vi "New Edit Element.vi"(8 "error in (no error)":errorcluster, 11 "Component-B in":refnum<class "Component-B.lvclass">) -> (0 "error out":errorcluster, 3 "Component-B out":refnum<class "Component-B.lvclass">)   [LabVIEW 2018, in "Component-B.lvclass"]
uses:
  Component-B.lvclass
  <vilib>/Utility/error.llb/Error Cluster From Error Code.vi
  <vilib>/ErrorRing/Error Ring.xnode
  U:/modules/labview-orm/demo/Component.lvclass
  U:/modules/labview-orm/_Serializable Base Object/_ISerializable.lvclass
panel:
  in  "Color":u32(colorbox)
  in  "cancel button":bool
  in  "ok button":bool
  in  "isObsolete":bool
  in  "status":u8
  in  "isEssencial_":bool
  in  "owner":string
  in  "RelatedIssues":dbl format="%.5g"
  out "uid":u64
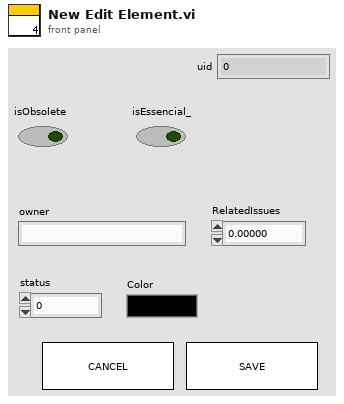
[diagram p1: front panel]
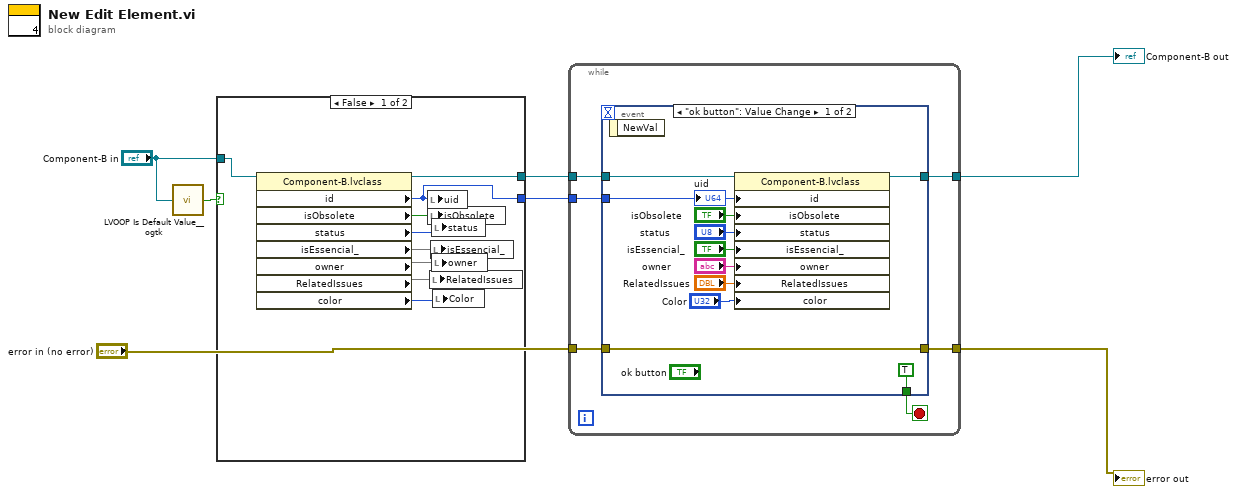
[diagram p0: block diagram]
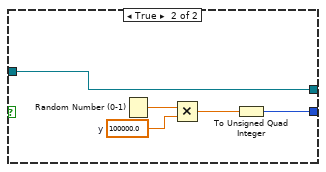
[diagram p2: hidden frame]
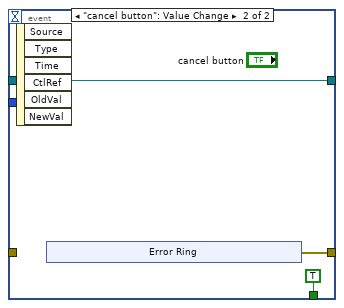
[diagram p3: hidden frame]
diagram:
  n1 = call <userlib>:"LVOOP Is Default Value__ogtk.vi"("Object"="Component-B in") -> ("Is Default Value?"=w2:bool)
  n2 = case shown="False" w2 {
    tunnel: [w14 w18] -> w7
    tunnel: "Component-B in" -> [w16 w17]
    tunnel: [w15 w17] -> w1
    frame False {
      n3 = property class="Component-B.lvclass"(reference=w16) -> (reference out=w15:refnum<class "Component-B.lvclass">, "id"=w14:i32, "isObsolete"=w8:bool, "status"=w9:u8, "isEssencial_"=w10, "owner"=w11, "RelatedIssues"=w12, "color"=w13:u32)  [unwired: 1 in, 1 out]
      n4 = local write "uid"(w14) -> ()
      n5 = local write "isObsolete"(w8) -> ()
      n6 = local write "RelatedIssues"(w12) -> ()
      n7 = local write "isEssencial_"(w10) -> ()
      n8 = local write "status"(w9) -> ()
      n9 = local write "owner"(w11) -> ()
      n10 = local write "Color"(w13) -> ()
    }
    frame True {
      w20 = 100000.0  # y
      n11 = Random Number (0-1)() -> (number: 0 to 1=w21:dbl)
      n12 = Multiply(x=w21, y=w20) -> (x*y=w19:dbl)
      n13 = To Unsigned Quad Integer(1:w19) -> (0:w18:u64)
    }
  }
  n14 = while {
    tunnel: "error in (no error)" -> [w24]
    tunnel: w1 -> [w27]
    tunnel: [w26] -> w4
    tunnel: [w25] -> w5
    tunnel: w7 -> [w22]
    stop <- w23 stop-if-true
    n15 = event shown="[0] \"ok button\": Value Change" {
      selector: _ -> [_ _]
      dyn-events: _ -> [_ _]
      timeout: _ -> [_ _]
      tunnel: w27 -> [w38 w41]
      tunnel: [w37 w41] -> w26
      tunnel: [w36 w40] -> w25
      tunnel: w24 -> [w36 _]
      tunnel: [TRUE TRUE] -> w23
      tunnel: w22 -> [w34 _]
      event "ok button": Value Change {
        n16 = event-data() -> ()  [unwired: 1 in, 1 out]
        n17 = property class="Component-B.lvclass"(reference=w38, "id"=w34, "isObsolete"="isObsolete", "status"="status", "isEssencial_"="isEssencial_", "owner"="owner", "RelatedIssues"="RelatedIssues", "color"="Color") -> (reference out=w37:refnum<class "Component-B.lvclass">)  [unwired: 1 in, 1 out]
        "uid" <- w34
      }
      event "cancel button": Value Change {
        n18 = event-data() -> ()  [unwired: 1 in, 6 out]
        n19 = xnode "Error Ring"() -> ("error out"=w40:errorcluster)
      }
    }
  }
  "error out" <- w5
  "Component-B out" <- w4
